vi "RT Driver VI.vi"(6 "Device Clock":string, 9 "Device Inputs FIFO":refnum<k33>, 10 "Device Outputs FIFO":refnum<k33>, 11 "Device Reference":T1 format="%.0x") -> ()   [LabVIEW 2014, in "CAN Bus Monitor Engine.lvlib"]
uses:
  CAN Bus Monitor Engine.lvlib
  <vilib>/NI Veristand/Custom Device API/Custom Device Item Ref.ctl
  <vilib>/NI Veristand/Custom Device API/Custom Device Channel Type.ctl
  Controls/XNET Communication Properties.ctl
  Controls/CAN IO Mode.ctl
  Controls/Analyze Array.ctl
  Controls/FlexRay Channel.ctl
  Controls/XNET BM Frame.ctl
  Shared/Constants.vi
  <vilib>/NI Veristand/Custom Device API/Get Item Property (String).vi
  <vilib>/NI Veristand/Custom Device API/Get Item Property (U32).vi
  <vilib>/NI Veristand/Custom Device API/Custom Device API.lvlib
  <vilib>/NI Veristand/Custom Device Tools/Custom Device Utility Library/Custom Device Utility Library.lvlib
  Shared/CAN Bus Monitor Shared.lvlib
panel:
  in  "Initialization Status Notifier":refnum<notifier>
  in  "Status Notifier":refnum<notifier>
  # "Custom Device Template\nv1.0"
  # "Use this template as a starting point for creating a custom device code module. The input controls shown here are specially named controls that the system will use to provide the device loop with data. The controls are not required for the device loop to run. For instance, if the device doesn't produce any output data, then you don't need the Device Outputs FIFO control. If you do use these controls, however, they need to have these exact names to be functional."
  # "The optional status notifier element is used to notify the RT engine of the last state of the custom device, and to indicate the device has completed execution. If this control is not used, a default No Error value is returned to the system when the device finishes execution.\n\nNote: This error state is not checked until the system shuts down. Use an output status channel to send more immediate status values to the system."
  # "This optional input can be used to send the VeriStand Engine the final status of the custom device initalization process. If this control exists on the custom device front panel, the VeriStand Engine will wait for a status update before starting up. If the custom device reports an error, that will abort the execution of the current configuration in the VeriStand Engine.\n\nThis control can be deleted if the custom device does not need to send the initialization status update."
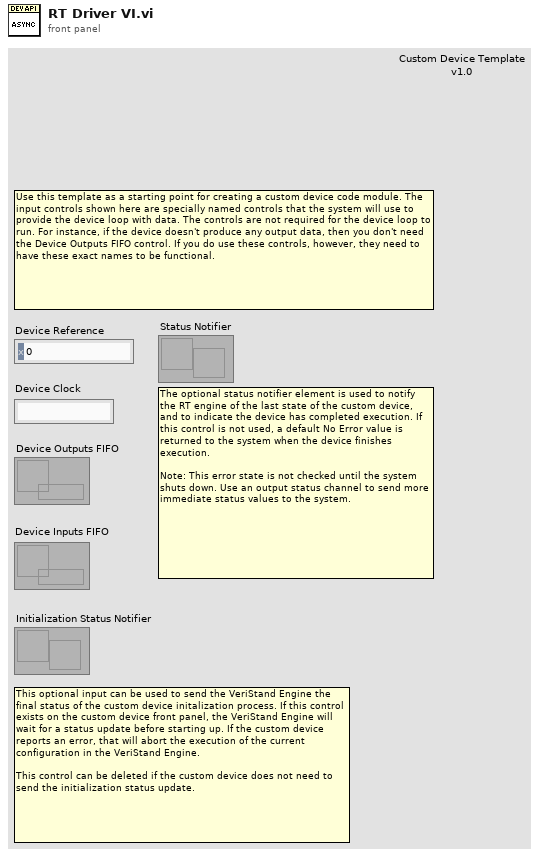
[diagram p1: front panel]
types:
  T1 = typedef "Custom Device API.lvlib/Custom Device Item Ref.ctl" = u64
  T2 = typedef "CAN Bus Monitor Engine.lvlib/XNET Communication Properties.ctl" = cluster{"Port Name":string, "Baud Rate":u32, "CAN I/O Mode":T3, "XNET Session":refnum<k21>}
  T3 = typedef "CAN Bus Monitor Engine.lvlib/CAN IO Mode.ctl" = u32
  T4 = typedef "Custom Device API.lvlib/Custom Device Channel Type.ctl" = enum16{"Input", "Output"}
  T5 = typedef "CAN Bus Monitor Engine.lvlib/Analyze Array.ctl" = cluster{"# Rx Frames":u32, "Last Timestamp":timestamp, "RateInc":dbl, "# Frames per Rate":u32, "MessageName":string, "Cycle Number":u32, "FlexRay Channel":T6, "Message Comment":string, "CAN frame In":T7}[]
  T6 = typedef "CAN Bus Monitor Engine.lvlib/FlexRay Channel.ctl" = u16
  T7 = typedef "CAN Bus Monitor Engine.lvlib/XNET BM Frame.ctl" = cluster{"timestamp":timestamp, "payload":u8[], "identifier / slot":u32, "Data type":u8, "payload length":u8, "CAN":cluster{"extended?":bool}, "FlexRay":cluster{"cycle count":u8, "startup?":bool, "sync?":bool, "preamble?":bool, "ch A":bool, "ch B":bool, "macrotick":u16}, "echo?":bool}
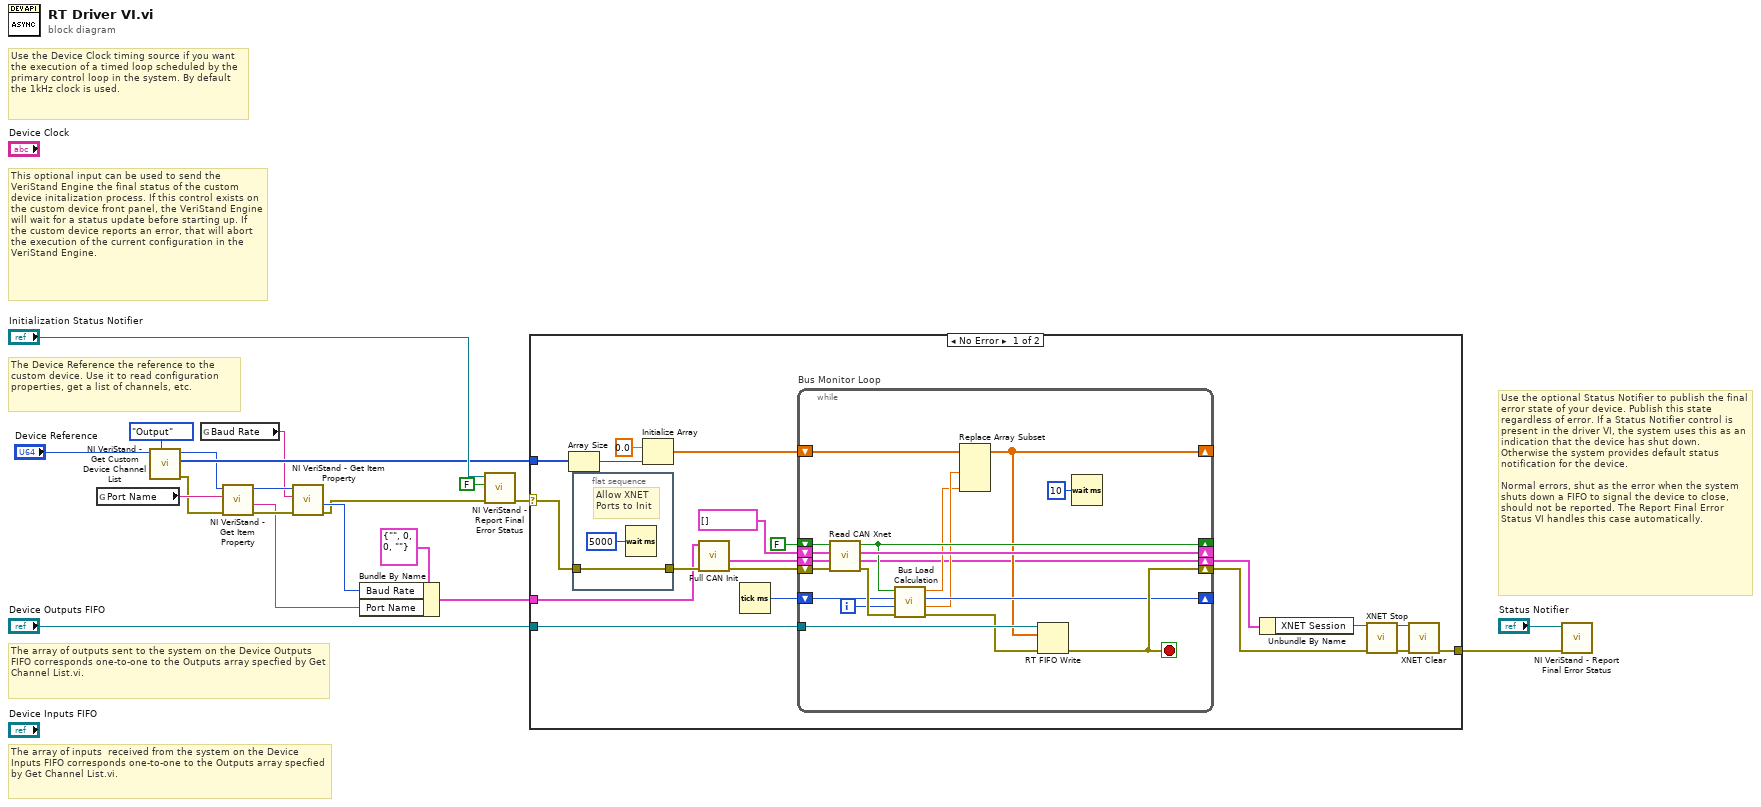
[diagram p0: block diagram]
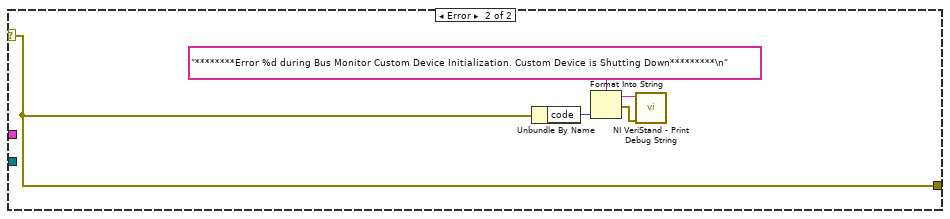
[diagram p2: hidden frame]
diagram:
  # "This optional input can be used to send the VeriStand Engine the final status of the custom device initalization process. If this control exists on the custom device front panel, the VeriStand Engine will wait for a status update before starting up. If the custom device reports an error, that will abort the execution of the current configuration in the VeriStand Engine."
  # "The array of inputs  received from the system on the Device Inputs FIFO corresponds one-to-one to the Outputs array specfied by Get Channel List.vi."
  # "Use the optional Status Notifier to publish the final error state of your device. Publish this state regardless of error. If a Status Notifier control is present in the driver VI, the system uses this as an indication that the device has shut down. Otherwise the system provides default status notification for the device.\n\nNormal errors, shut as the error when the system shuts down a FIFO to signal the device to close, should not be reported. The Report Final Error Status VI handles this case automatically."
  # "The array of outputs sent to the system on the Device Outputs FIFO corresponds one-to-one to the Outputs array specfied by Get Channel List.vi."
  # "The Device Reference the reference to the custom device. Use it to read configuration properties, get a list of channels, etc."
  # "Use the Device Clock timing source if you want the execution of a timed loop scheduled by the primary control loop in the system. By default the 1kHz clock is used."
  n1 = global read "Constants.vi" "Port Name"() -> (w13:string)
  n2 = call <vilib>:"NI VeriStand - Get Custom Device Channel List.vi"("Channel Type"=Custom_Device_Channel_Type."Output", "Device Ref in"="Device Reference") -> ("error out"=w11:errorcluster, "Specified Channel Ref List"=w17:T1[], "Device Ref out"=w10:T1)  [unwired: 1 in, 6 out]
  n3 = global read "Constants.vi" "Baud Rate"() -> (w7:string)
  n4 = call-poly <vilib>:"NI VeriStand - Get Item Property.vi"("error in (no error)"=w11, "Property Name"=w13, "Item Ref in"=w10) -> ("error out"=w8:errorcluster, "Value"=w5:string, "Item Ref out"=w9:T1)  [unwired: 5 in, 1 out]
  n5 = call-poly <vilib>:"NI VeriStand - Get Item Property.vi"("error in (no error)"=w8, "Property Name"=w7, "Item Ref in"=w9) -> ("error out"=w3:errorcluster, "Value"=w6:u32)  [unwired: 5 in, 2 out]
  n6 = Bundle By Name(cluster=T2 {"Port Name"="", "Baud Rate"=0, "CAN I/O Mode"=0, "XNET Session"=""}, "Baud Rate"=w6, "Port Name"=w5) -> (w4:T2)
  n7 = call <vilib>:"NI VeriStand - Report Final Error Status.vi"("error in (no error)"=w3, "Filter FIFO & Shutdown Errors (T)"=FALSE ("Filter FIFO Errors (T)"), "Status Notifier"="Initialization Status Notifier") -> ("error out"=w15:errorcluster)  [unwired: 8 out]
  n8 = case shown="No Error" w15 {
    selector: w15 -> [w34 w64]
    tunnel: "Device Outputs FIFO" -> [w39 _]
    tunnel: w17 -> [w35 _]
    tunnel: [w26 w64] -> w2
    tunnel: w4 -> [w24 _]
    frame No Error {
      n9 = Array Size(array=w35) -> (size(s)=w36:i32)
      n10 = flat-sequence {
        tunnel: w34 -> [w41]
        tunnel: [w41] -> w25
        frame #0 {
          # "Allow XNET\nPorts to Init"
          n11 = Wait (ms)(milliseconds to wait=u32 5000) -> ()  [unwired: 1 out]
        }
      }
      n12 = Initialize Array(0.0 ("element"), w36) -> (w37:dbl[])
      n13 = call "Full CAN Init.vi"("error in (no error)"=w25, "XNET Commuication Properties"=w24) -> ("error out"=w23:errorcluster, "XNET Communication Properties Out"=w22:T2)  [unwired: 8 in]
      n14 = Tick Count (ms)() -> (millisecond timer value=w32:u32)
      n15 = while "Bus Monitor Loop" {
        shift-right: [w58] -> w27
        shift-left: w23 -> [w56]
        shift-right: [w44] -> _
        shift-left: w37 -> [w47]
        tunnel: w39 -> [w60]
        shift-right: [w52] -> _
        shift-left: FALSE ("NewData out") -> [w55]
        shift-right: [w42] -> w28
        shift-left: w22 -> [w43]
        shift-right: [w53] -> _
        shift-left: T5 [] ("Data Array") -> [w54]
        shift-right: [w48] -> _
        shift-left: w32 -> [w51]
        i -> [w50]
        stop <- w58 stop-if-true
        n16 = call "Read CAN Xnet.vi"("error in"=w56, "XNET Communications Properties"=w43, "Tlg Data Array"=w54, "NewData In"=w55) -> ("error out"=w57:errorcluster, "XNET Communications Properties Out"=w42:T2, "Tlg Data Array out"=w53:T5, "NewData"=w52:bool)
        n17 = call "Bus Load Calculation.vi"("error in"=w57, "Current Iteration"=w50, "millisecond timer value in"=w51, "NewData"=w52) -> ("error out"=w49:errorcluster, "BusLoad"=w46:dbl, "millisecond timer value out"=w48:u32, "Peak Bus Load"=w45:dbl)  [unwired: 4 in]
        n18 = Replace Array Subset(array=w47, new element #1=w46, new element #2=w45) -> (w44:dbl[])  [unwired: 2 in]
        n19 = RT FIFO Write(0:w60, 1:w44, 3:w49) -> (11:w58:errorcluster)  [unwired: 1 in, 4 out]
        n20 = Wait (ms)(milliseconds to wait=u32 10) -> ()  [unwired: 1 out]
      }
      n21 = Unbundle By Name(w28) -> ("XNET Session"=w29:refnum<k21>)
      n22 = call <vilib>:"XNET Stop.vi"("session in"=w29, "error in (no error)"=w27) -> ("session out"=w30:refnum<k21>, "error out"=w31:errorcluster)  [unwired: 12 in]
      n23 = call <vilib>:"XNET Clear.vi"("session in"=w30, "error in (no error)"=w31) -> ("error out"=w26:errorcluster)  [unwired: 13 in]
    }
    frame Error {
      n24 = Unbundle By Name(w64) -> ("code"=w63:i32)
      n25 = Format Into String(format string="********Error %d during Bus Monitor Custom Device Initialization. Custom Device is Shutting Down*********\n", w63) -> (resulting string=w62:string, error out=w61:errorcluster)  [unwired: 2 in]
      n26 = call <vilib>:"NI VeriStand - Print Debug String.vi"("error in (no error)"=w61, "Message"=w62) -> ()  [unwired: 9 in, 1 out]
    }
  }
  n27 = call <vilib>:"NI VeriStand - Report Final Error Status.vi"("error in (no error)"=w2, "Status Notifier"="Status Notifier") -> ()  [unwired: 1 in, 9 out]
